vi "Manipulate_Table.vi"(3 "Table size":i32=200000, 4 "Latest Row":dbl[](array[numeric]) format="%.2f", 5 "Table Input":dbl[][](array[numeric]) format="%.2f") -> (0 "History length":i32=200, 2 "Table Output":dbl[][](array[numeric]) format="%.2f")   [LabVIEW 2020]
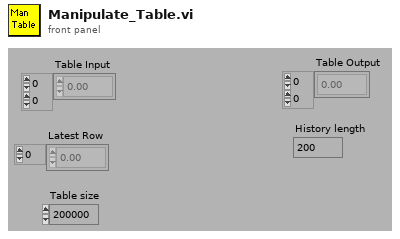
[diagram p1: front panel]
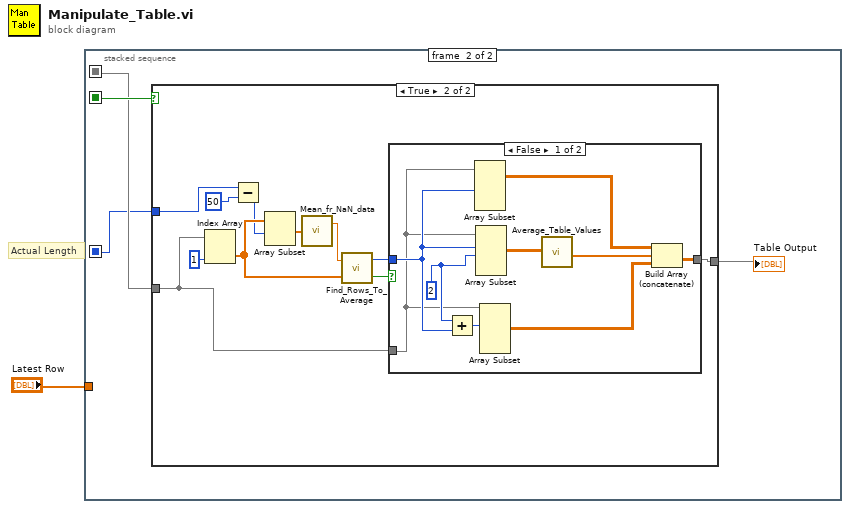
[diagram p0: block diagram]
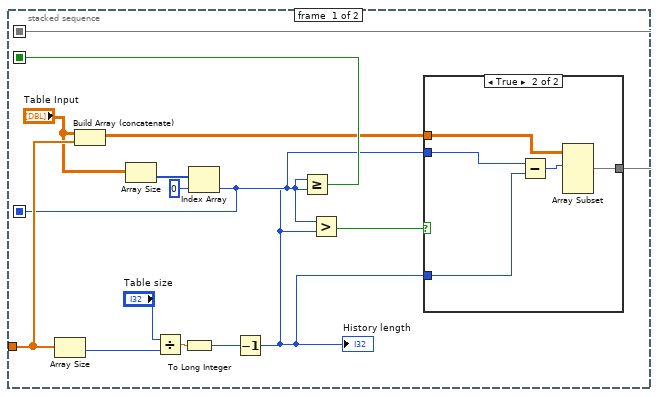
[diagram p2: hidden frame]
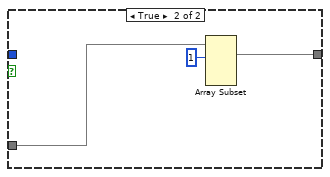
[diagram p5: hidden frame]
diagram:
  # "Actual Length"
  n1 = stacked-sequence {
    seq-local: [w11 _] -> [_ w25]
    seq-local: [w8 _] -> [_ w24]
    seq-local: [w4 _] -> [_ w22]
    tunnel: "Latest Row" -> [w9 _]
    frame #0 {
      n2 = Array Size(array=w9) -> (size(s)=w14:i32)
      n3 = Build Array (concatenate)("Table Input", w9) -> (w7:dbl[][])
      n4 = Array Size(array="Table Input") -> (size(s)=w13:i32[])
      n5 = Divide(x="Table size", y=w14) -> (x/y=w15:dbl)
      n6 = To Long Integer(number=w15) -> (32bit integer=w5:i32)
      n7 = Index Array(array=w13, index=0) -> (element=w4:i32)
      n8 = Decrement(x=w5) -> (x-1=w3:i32)
      "History length" <- w3
      n9 = Greater Or Equal?(x=w4, y=w3) -> (x >= y?=w11:bool)
      n10 = Greater?(x=w4, y=w3) -> (0:w10:bool)
      n11 = case shown="True" w10 {
        tunnel: w7 -> [w16 w19]
        tunnel: w4 -> [_ w18]
        tunnel: w3 -> [_ w17]
        tunnel: [w16 w20] -> w8
        frame False {
        }
        frame True {
          n12 = Subtract(x=w18, y=w17) -> (x-y=w21:i32)
          n13 = Array Subset(array=w19, index (row)=w21) -> (w20:dbl[][])  [unwired: 3 in]
        }
      }
    }
    frame #1 {
      n14 = case shown="True" w25 {
        tunnel: w24 -> [w26 w34]
        tunnel: [w26 w33] -> w23
        tunnel: w22 -> [_ w32]
        frame False {
        }
        frame True {
          n15 = Index Array(array=w34, index (col)=1 ("Index")) -> (element=w30:dbl[])  [unwired: 1 in]
          n16 = Subtract(x=w32, y=50) -> (x-y=w29:i32)
          n17 = Array Subset(array=w30, index=w29) -> (w28:dbl[])  [unwired: 1 in]
          n18 = call "Mean_fr_NaN_data.vi"("Data"=w28) -> ("Mean value"=w27:dbl)  [unwired: 1 out]
          n19 = call "Find_Rows_To_Average.vi"("Averaging Period"=w30, "Approx Scan Period"=w27) -> ("Remove top Row"=w37:bool, "Index"=w36:i32)
          n20 = case shown="False" w37 {
            tunnel: w34 -> [w42 w49]
            tunnel: [w38 w48] -> w33
            tunnel: w36 -> [w45 _]
            frame False {
              w46 = 2 ("Array Length")
              n21 = Add(x=w46, y=w45) -> (x+y=w44:i32)
              n22 = Array Subset(array=w42, length (row)=w45) -> (w39:dbl[][])  [unwired: 3 in]
              n23 = Array Subset(array=w42, index (row)=w45, length (row)=w46) -> (w43:dbl[][])  [unwired: 2 in]
              n24 = Array Subset(array=w42, index (row)=w44) -> (w41:dbl[][])  [unwired: 3 in]
              n25 = call "Average_Table_Values.vi"("Table values to average"=w43) -> ("Averaged Row"=w40:dbl[])
              n26 = Build Array (concatenate)(w39, w40, w41) -> (w38:dbl[][])
            }
            frame True {
              n27 = Array Subset(array=w49, index (row)=1 ("Array Index")) -> (w48:dbl[][])  [unwired: 3 in]
            }
          }
        }
      }
      "Table Output" <- w23
    }
  }
